vi "testV4.vi"() -> ()   [LabVIEW 2020]
uses:
  <vilib>/DAQmx/read.llb/DAQmx Read (Analog 2D DBL NChan NSamp).vi
  <vilib>/Analysis/baseanly.llb/Mean (DBL).vi
  <vilib>/DAQmx/miscellaneous.llb/DAQmx Fill In Error Info.vi
  <vilib>/Analysis/NI_AALBase.lvlib
  <resource>/objmgr/daqmx.rc
panel:
  in  "Table":string[][](table)
  out "text":string
  out "transposed array":dbl[][](array[numeric])
  out "size(s)":i32
  out "x/y":dbl
  in  "Sampling Time":u32=5
  in  "DAQmx Task Name 2":refnum<k21>="MyTemperatureTask"
  in  "Read Time (s) 2":u32=60
  out "Array":dbl[][](array[numeric])
  in  "stop":bool
  out "F-format string":string[](array[string])
  in  "Path":path=path "E:/KMUTT/Master Degree/labviewjgsee/log"
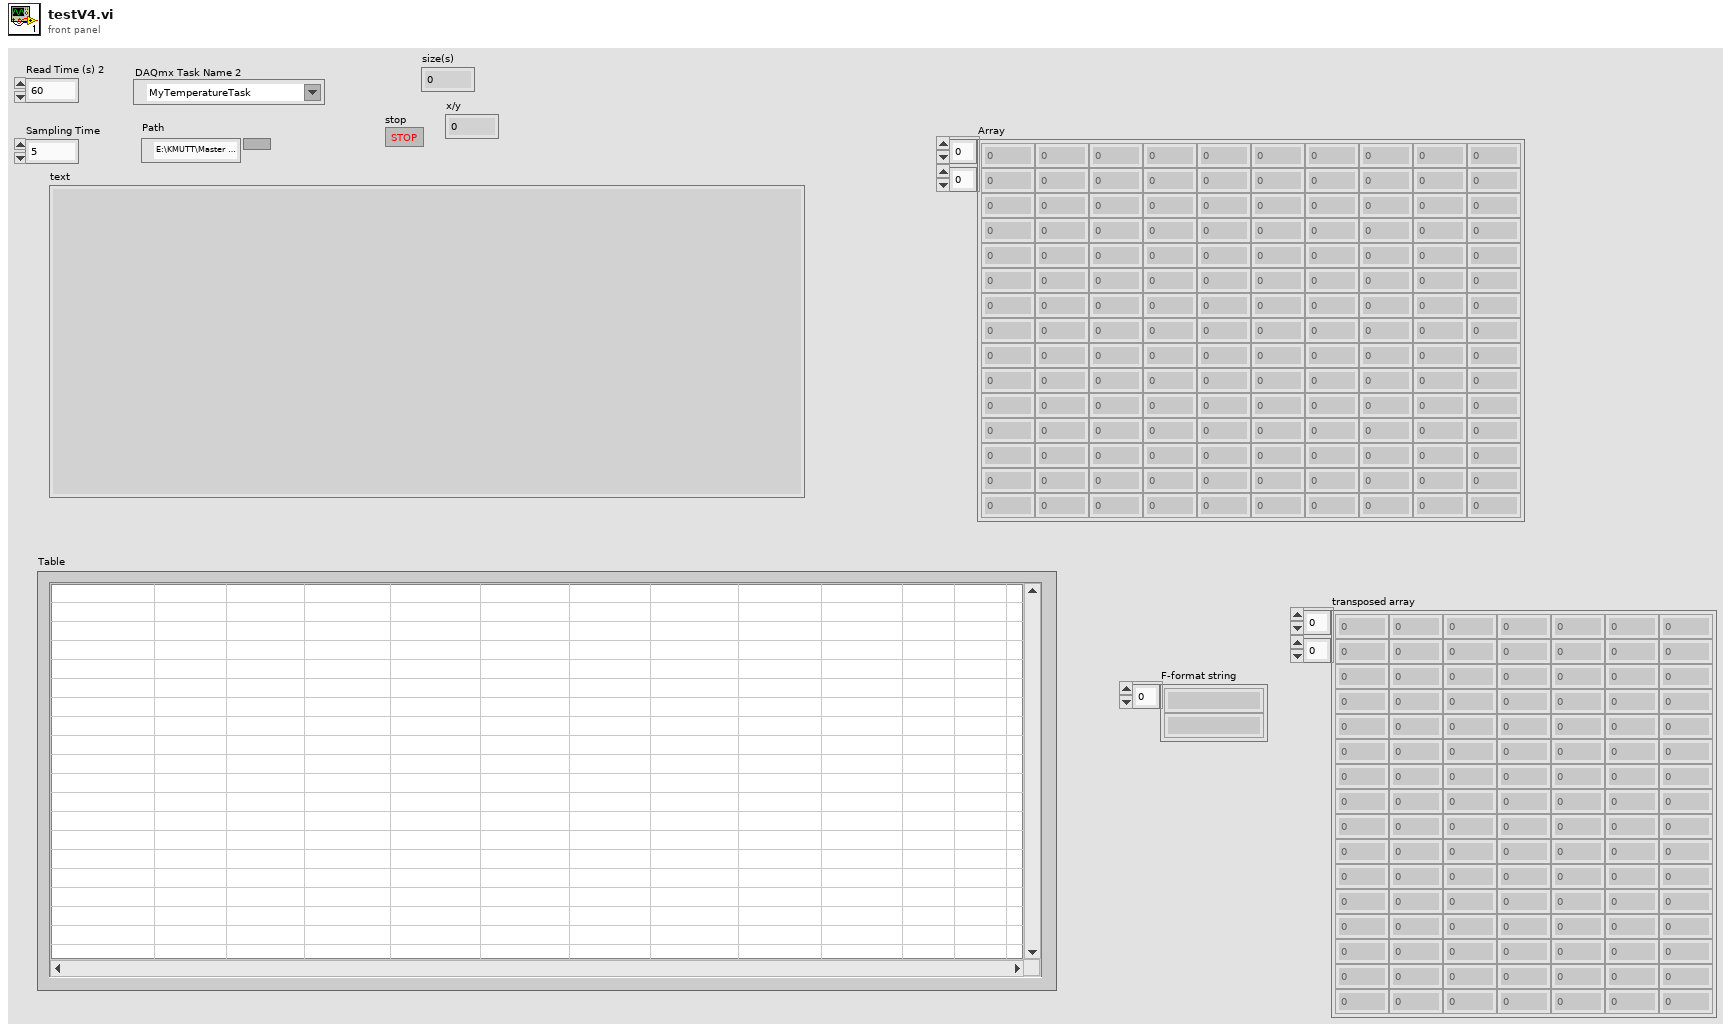
[diagram p1: front panel]
types:
  T1 = enum16{"open", "replace", "create", "open or create", "replace or create", "replace or create with confirmation"}
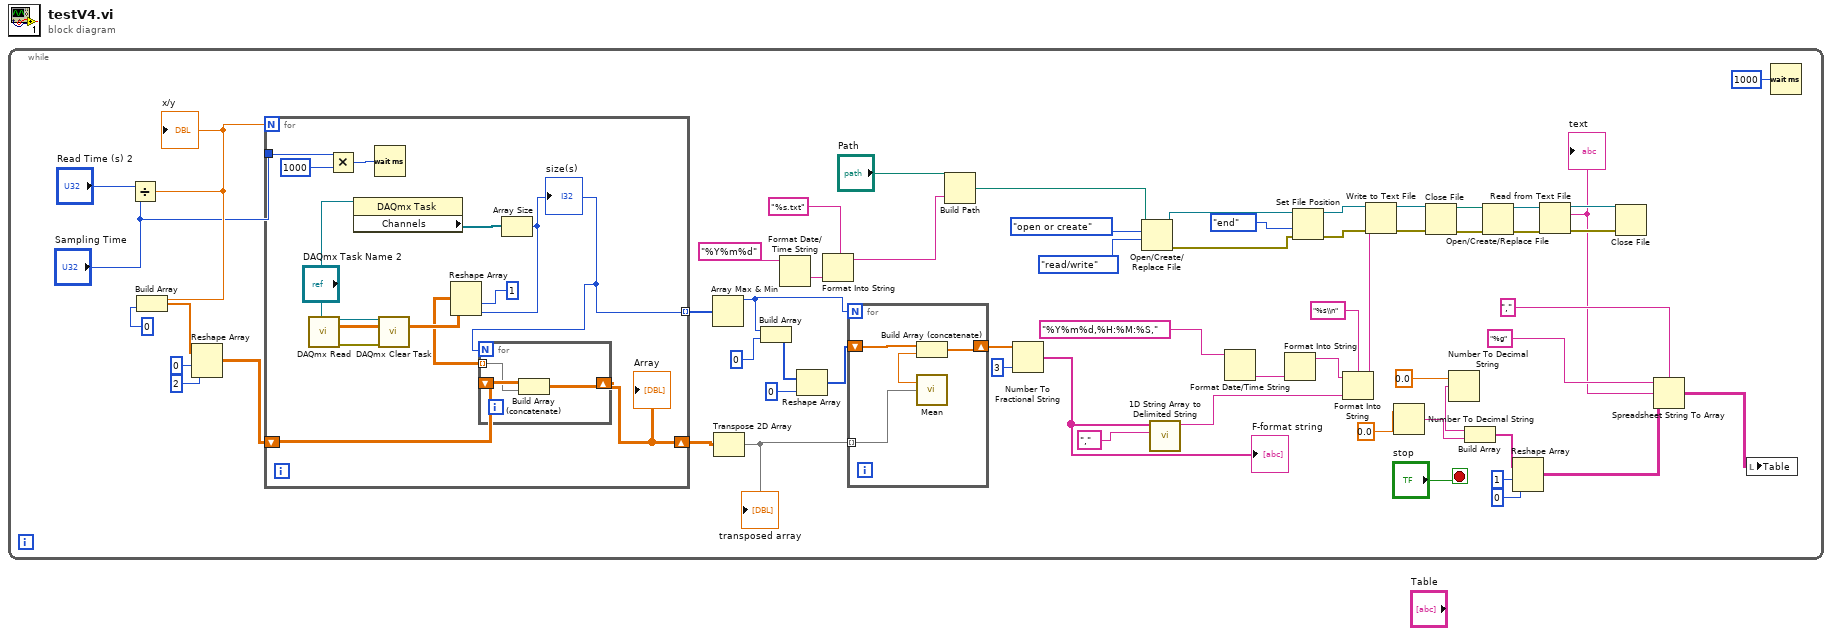
[diagram p0: block diagram]
diagram:
  n1 = while {
    stop <- "stop" stop-if-true
    n2 = Divide(x="Read Time (s) 2", y="Sampling Time") -> (x/y=w34:dbl)
    "x/y" <- w34
    n3 = Build Array(w34, 0 ("element")) -> (w39:dbl[])
    n4 = Reshape Array(w39, 0 ("dimension size"), 2 ("dimension size")) -> (w36:dbl[][])
    n5 = for {
      N: w34 -> [_]
      shift-right: [w69] -> w31
      shift-left: w36 -> [w68]
      tunnel: "Sampling Time" -> [w67]
      tunnel: [w62] -> w32 mode=indexing
      n6 = call-poly <vilib>:"DAQmx Read.vi"("task/channels in"="DAQmx Task Name 2") -> ("task out"=w73:refnum<k21>, "data"=w71:dbl[][], "error out"=w74:errorcluster)  [unwired: 12 in]
      n7 = Multiply(x=w67, y=u32 1000) -> (x*y=w65:u32)
      n8 = property class="DAQmx Task"(reference="DAQmx Task Name 2") -> ("Channels"=w64:refnum<k21>[])  [unwired: 1 in, 2 out]
      n9 = Wait (ms)(milliseconds to wait=w65) -> ()  [unwired: 1 out]
      n10 = call <vilib>:"DAQmx Clear Task.vi"("task in"=w73, "error in"=w74) -> ()  [unwired: 13 in, 1 out]
      n11 = Array Size(array=w64) -> (size(s)=w62:i32)
      "size(s)" <- w62
      n12 = Reshape Array(w71, 1 ("dimension size"), w62) -> (w70:dbl[][])
      n13 = for {
        N: w62 -> [_]
        shift-right: [w76] -> w69
        shift-left: w68 -> [w77]
        tunnel: w70 -> [w75] mode=indexing
        n14 = Build Array (concatenate)(w77, w75) -> (w76:dbl[][])
      }
      "Array" <- w69
    }
    n15 = Array Max & Min(array=w32) -> (max value=w28:i32)  [unwired: 3 out]
    n16 = Transpose 2D Array(2D array=w31) -> (transposed array=w30:dbl[][])
    "transposed array" <- w30
    n17 = Build Array(w28, 0 ("element")) -> (w26:i32[])
    n18 = Format Date/Time String(time format string (%c)="%Y%m%d") -> (date/time string=w52:string)  [unwired: 2 in]
    n19 = Reshape Array(w26, 0 ("dimension size")) -> (w25:i32[])
    n20 = Format Into String(format string="%s.txt", w52) -> (resulting string=w49:string)  [unwired: 2 in, 1 out]
    n21 = for {
      N: w28 -> [_]
      tunnel: w30 -> [w81] mode=indexing
      shift-right: [w79] -> w41
      shift-left: w25 -> [w78]
      n22 = call-poly <vilib>:"Mean.vi"("X"=w81) -> ("mean"=w80:dbl)  [unwired: 1 out]
      n23 = Build Array (concatenate)(w78, w80) -> (w79:dbl[])
    }
    n24 = Build Path(base path="Path", name or relative path=w49) -> (appended path=w48:path)
    n25 = Number To Fractional String(number=w41, precision (6)=i16 3) -> (F-format string=w42:string[])  [unwired: 2 in]
    "F-format string" <- w42
    n26 = Open/Create/Replace File(file path (use dialog)=w48, operation (0:open)=T1."open or create", access (0:read/write)=enum16{"read/write", "read-only", "write-only"}."read/write") -> (refnum out=w23:refnum<file>, error out=w56:errorcluster)  [unwired: 3 in, 1 out]
    n27 = call <vilib>:"1D String Array to Delimited String.vi"("delimiter"="," ("format string"), "string array"=w42) -> ("delimited string"=w47:string)  [unwired: 9 in]
    n28 = Format Date/Time String(time format string (%c)="%Y%m%d,%H:%M:%S,") -> (date/time string=w44:string)  [unwired: 2 in]
    n29 = Format Into String(w44) -> (resulting string=w43:string)  [unwired: 3 in, 1 out]
    n30 = Set File Position(refnum=w23, from (0:start)=enum16{"start", "end", "current"}."end", error in=w56) -> (refnum out=w57:refnum<file>, error out=w55:errorcluster)  [unwired: 1 in]
    n31 = Format Into String(format string="%s\\n", initial string=w43, w47) -> (resulting string=w15:string)  [unwired: 1 in, 1 out]
    n32 = Write to Text File(file (use dialog)=w57, text=w15, error in=w55) -> (refnum out=w22:refnum<file>, error out=w21:errorcluster)  [unwired: 1 in, 1 out]
    n33 = Number To Decimal String(number=0.0 ("element")) -> (decimal integer string=w2:string)  [unwired: 1 in]
    n34 = Close File(refnum=w22, error in=w21) -> (path=w20:path, error out=w19:errorcluster)
    n35 = Number To Decimal String(number=0.0 ("element")) -> (decimal integer string=w4:string)  [unwired: 1 in]
    n36 = Build Array(w4, w2) -> (w7:string[])
    n37 = Open/Create/Replace File(file path (use dialog)=w20, error in=w19) -> (refnum out=w18:refnum<file>, error out=w17:errorcluster)  [unwired: 4 in, 1 out]
    n38 = Reshape Array(w7, 1 ("dimension size"), 0 ("dimension size")) -> (w8:string[][])
    n39 = Read from Text File(file (use dialog)=w18, error in=w17) -> (refnum out=w16:refnum<file>, text=w11:string, error out=w12:errorcluster)  [unwired: 2 in, 1 out]
    "text" <- w11
    n40 = Close File(refnum=w16, error in=w12) -> ()  [unwired: 2 out]
    n41 = Spreadsheet String To Array(delimiter (Tab)=",", format string="%g", spreadsheet string=w11, array type (2D Dbl)=w8) -> (array=w6:string[][])
    n42 = local write "Table"(w6) -> ()
    n43 = Wait (ms)(milliseconds to wait=u32 1000) -> ()  [unwired: 1 out]
  }
